vi "TX Timeout.vi"(2 "error in (no error)":errorcluster) -> (4 "error out":errorcluster)   [LabVIEW 2021, in "CAN_Logic.lvclass"]
uses:
  CAN_Logic.lvclass
  CAN_Logic.lvclass/CAN_Logic.ctl
  typedef/Error Global.vi
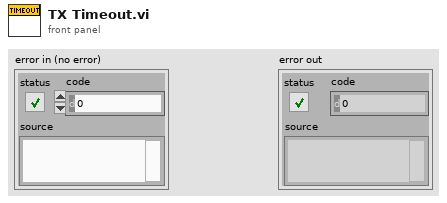
[diagram p1: front panel]
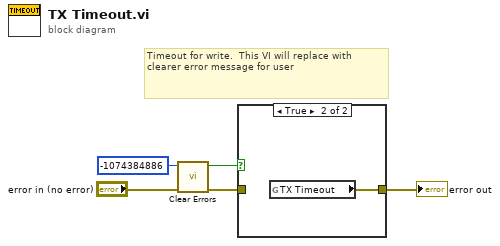
[diagram p0: block diagram]
diagram:
  # "Timeout for write.  This VI will replace with clearer error message for user"
  n1 = call <vilib>:"Clear Errors.vi"("error in (no error)"="error in (no error)", "specific error code to clear (0: all)"=-1074384886) -> ("error out"=w2:errorcluster, "specific error cleared?"=w3:bool)  [unwired: 4 in]
  n2 = case shown="True" w3 {
    tunnel: w2 -> [w6 _]
    tunnel: [w6 w7] -> w1
    frame False {
    }
    frame True {
      n3 = global read "Error Global.vi" "TX Timeout"() -> (w7:errorcluster)
    }
  }
  "error out" <- w1
